vi "001-MyFirstProject-MainVI.vi"() -> ()   [LabVIEW 2019]
panel:
  in  "Size:Width":u32
  in  "Visible":bool
  out "String":string
  out "Low Limit":bool
  out "High Limit":bool
  in  "Numeric":dbl
  out "Tank":dbl(slide) scale=0.0..10.0
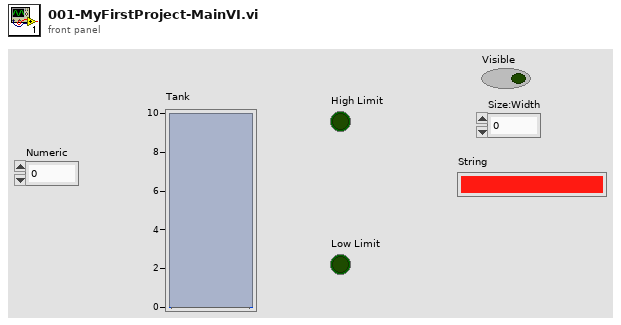
[diagram p1: front panel]
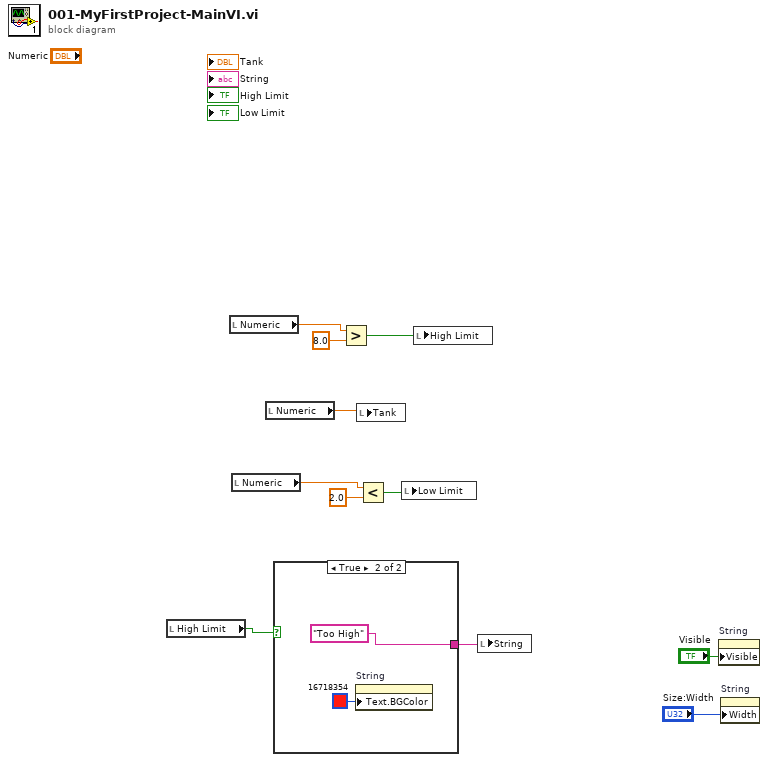
[diagram p0: block diagram]
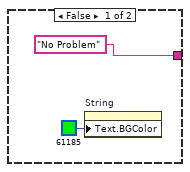
[diagram p2: hidden frame]
diagram:
  n1 = local read "High Limit"() -> (w3:bool)
  n2 = local read "Numeric"() -> (w6:dbl)
  n3 = local read "Numeric"() -> (w5:dbl)
  n4 = local read "Numeric"() -> (w7:dbl)
  n5 = case shown="True" w3 {
    tunnel: ["No Problem" ("String") "Too High" ("String")] -> w9
    frame False {
      n6 = property on="String" class="Str"("Text.BGColor"=u32 61185 ("Text.Text Colors:BG Color")) -> ()  [unwired: 2 in, 2 out]
    }
    frame True {
      n7 = property on="String" class="Str"("Text.BGColor"=u32 16718354 ("Text.Text Colors:BG Color")) -> ()  [unwired: 2 in, 2 out]
    }
  }
  n8 = Greater?(x=w6, y=8.0) -> (0:w4:bool)
  n9 = local write "Tank"(w7) -> ()
  n10 = Less?(x=w5, y=2.0) -> (x < y?=w8:bool)
  n11 = local write "Low Limit"(w8) -> ()
  n12 = local write "High Limit"(w4) -> ()
  n13 = local write "String"(w9) -> ()
  n14 = property on="String" class="Str"("Visible"="Visible") -> ()  [unwired: 2 in, 2 out]
  n15 = property on="String" class="Str"("Width"="Size:Width") -> ()  [unwired: 2 in, 2 out]
